vi "DS11202Z Init.vi"(0 "TestIndex":i32, 5 "S/DIV":T2(ring)=enum."1ms", 7 "存储深度":T1(ring), 9 "获取方式":enum16{"普通", "峰值", "平均", "高分辨率"}(ring)=enum."高分辨率", 11 "平均次数(2的n次方)":u16=2 min=2 step=2) -> (4 "OK?":bool, 15 "错误输出":errorcluster)   [LabVIEW 2015]
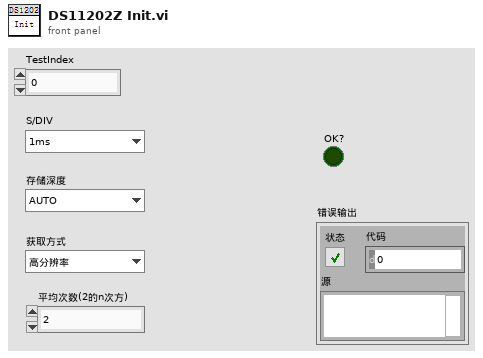
[diagram p1: front panel]
types:
  T1 = enum16{"AUTO", "12K", "120K", "1.2M", "12M", "24M"}
  T2 = enum16{"2ns", "5ns", "10ns", "20ns", "50ns", "100ns", "200ns", "500ns", "1us", "2us", "5us", "10us", "20us", "50us", "100us", "200us", "500us", "1ms", "2ms", "5ms", "10ms", "20ms", "50ms", "100ms", "200ms", "500ms", "1s", "2s", "5s", "10s", "20s"}
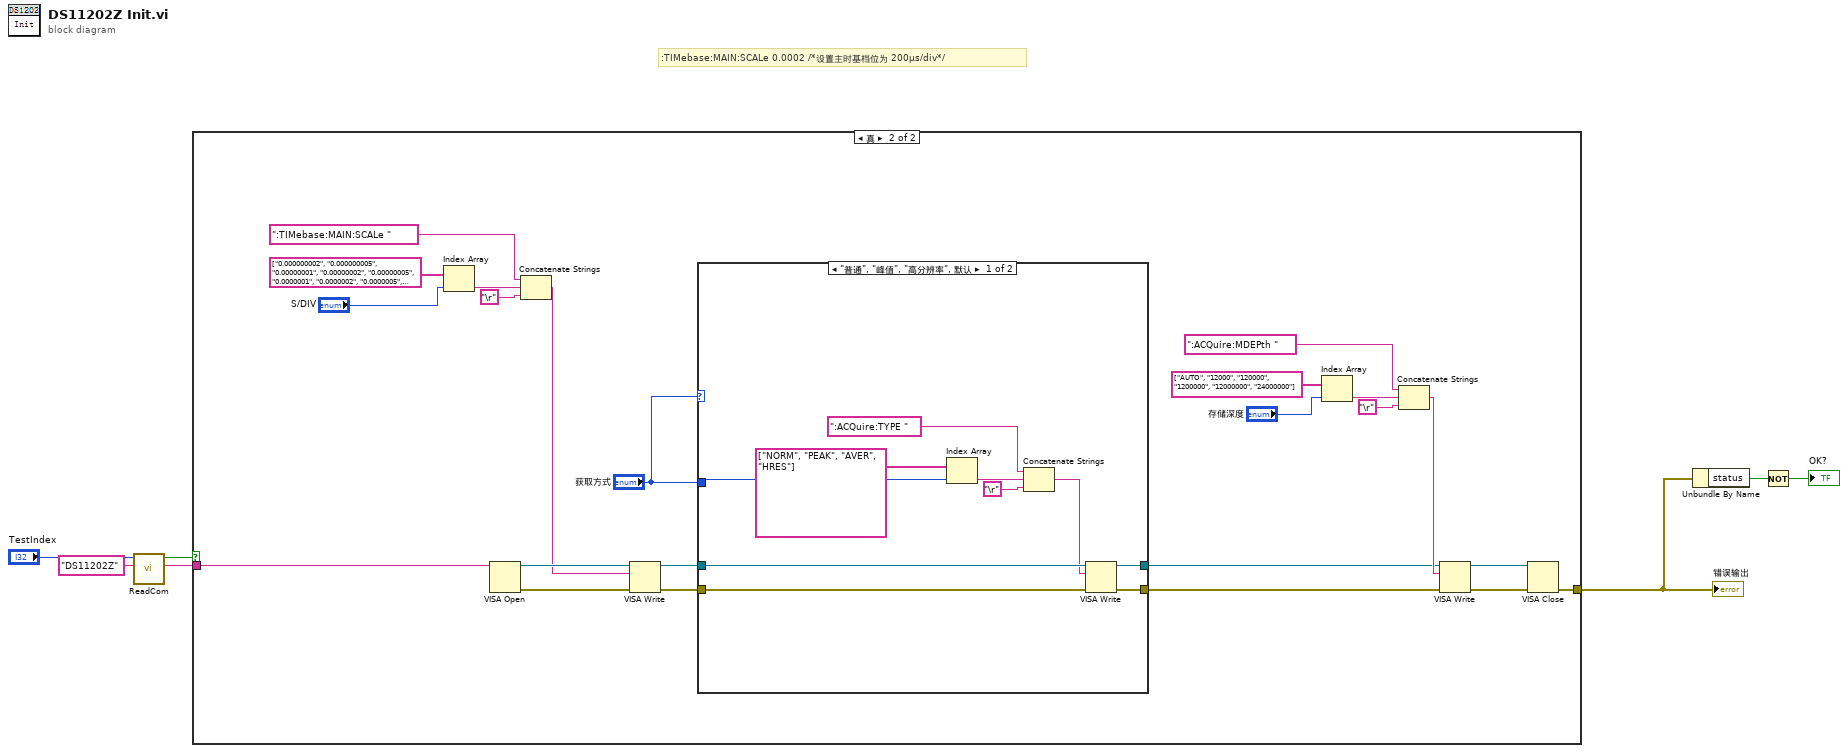
[diagram p0: block diagram]
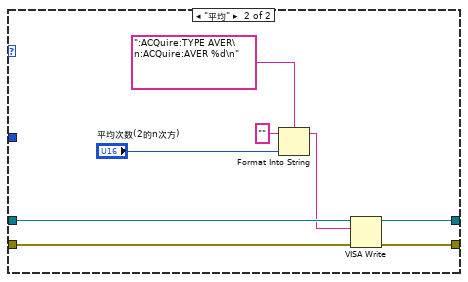
[diagram p3: hidden frame]
diagram:
  # ":TIMebase:MAIN:SCALe 0.0002 /*设置主时基档位为 200μs/div*/"
  n1 = call "ReadCom.vi"("仪器名称"="DS11202Z", "MyIndex"="TestIndex") -> ("COM"=w2:string, "OK?"=w1:bool)  [unwired: 7 in, 1 out]
  n2 = case shown="真" w1 {
    tunnel: [_ w9] -> w7
    tunnel: w2 -> [_ w8]
    frame False {
    }
    frame True {
      n3 = Index Array(array=string[] ["0.000000002", "0.000000005", "0.00000001", "0.00000002", "0.00000005", "0.0000001", "0.0000002", "0.0000005", "0.000001", "0.000002", "0.000005", "0.00001", "0.00002", "0.00005", "0.0001", "0.0002", "0.0005", "0.001", "0.002", "0.005", "0.01", "0.02", "0.05", "0.1", "0.2", "0.5", "1", "2", "5", "10", "20"], index="S/DIV") -> (element=w24:string)
      n4 = VISA Open(VISA resource name=w8) -> (VISA resource name=w30:refnum<visa-resource-name>, error out=w26:errorcluster)  [unwired: 1 in, 3 out]
      n5 = Concatenate Strings(":TIMebase:MAIN:SCALe " ("字符串"), w24, "\r") -> (w27:string)
      n6 = VISA Write(VISA resource name=w30, write buffer=w27, error in (no error)=w26) -> (VISA resource name out=w22:refnum<visa-resource-name>, error out=w14:errorcluster)  [unwired: 1 out]
      n7 = case shown="\"普通\", \"峰值\", \"高分辨率\", 默认" "获取方式" {
        tunnel: w22 -> [w34 w48]
        tunnel: "获取方式" -> [w32 _]
        tunnel: [w33 w47] -> w15
        tunnel: w14 -> [w35 w46]
        tunnel: [w36 w45] -> w13
        frame "普通", "峰值", "高分辨率", Default {
          n8 = Index Array(array=string[] ["NORM", "PEAK", "AVER", "HRES"], index=w32) -> (element=w39:string)
          n9 = Concatenate Strings(":ACQuire:TYPE " ("字符串"), w39, "\r") -> (w31:string)
          n10 = VISA Write(VISA resource name=w34, write buffer=w31, error in (no error)=w35) -> (VISA resource name out=w33:refnum<visa-resource-name>, error out=w36:errorcluster)  [unwired: 1 out]
        }
        frame "平均" {
          n11 = Format Into String(format string=":ACQuire:TYPE AVER\n:ACQuire:AVER %d\n" ("字符串"), initial string="" ("初始字符串"), "平均次数(2的n次方)") -> (resulting string=w41:string)  [unwired: 1 in, 1 out]
          n12 = VISA Write(VISA resource name=w48, write buffer=w41, error in (no error)=w46) -> (VISA resource name out=w47:refnum<visa-resource-name>, error out=w45:errorcluster)  [unwired: 1 out]
        }
      }
      n13 = Index Array(array=string[] ["AUTO", "12000", "120000", "1200000", "12000000", "24000000"], index="存储深度") -> (element=w20:string)
      n14 = Concatenate Strings(":ACQuire:MDEPth " ("字符串"), w20, "\r") -> (w17:string)
      n15 = VISA Write(VISA resource name=w15, write buffer=w17, error in (no error)=w13) -> (VISA resource name out=w11:refnum<visa-resource-name>, error out=w12:errorcluster)  [unwired: 1 out]
      n16 = VISA Close(VISA resource name=w11, error in (no error)=w12) -> (error out=w9:errorcluster)
    }
  }
  "错误输出" <- w7
  n17 = Unbundle By Name(w7) -> ("status"=w6:bool)
  n18 = Not(x=w6) -> (.not. x?=→"OK?":bool)
